vi "RSZVB Calibration Auto.vi"(0 "VISA session":refnum<visa-resource-name>, 1 "Channel (1)":i32=1, 2 "Calibration Kit Name":string, 5 "error in (no error)":errorcluster {"code" format="%.0x"}, 6 "Analyzer Port 1 (1)":i32=1, 7 "Cal Unit Port 1 (1)":i32=1, 8 "Analyzer Port 2 (1)":i32=1, 9 "Cal Unit Port 2 (1)":i32=1, 10 "Analyzer Port 3 (1)":i32=1, 11 "Cal Unit Port 3 (1)":i32=1, 12 "Analyzer Port 4 (1)":i32=1, 13 "Cal Unit Port 4 (1)":i32=1) -> (14 "dup VISA session":refnum<visa-resource-name>, 19 "error out":errorcluster {"code" format="%.0x"})   [LabVIEW 2011]
doc: "This VI selects and initiates a one-port, two-port, three-port or four-port automatic calibration at arbitrary analyzer and calibration unit ports.\n\nNote(s):\n\n(1) Port numbers of the analyzer:\nFor an n-port automatic calibration (n = 1 to 4), n arbitrary (not necessarily consecutive) port numbers must be specified.\n\n(2) Port numbers of the cal unit:\nFor an n-port automatic calibration (n = 1 to 4), n arbitrary (not necessarily consecutive) port numbers must be specified. It is possible to combine arbitrary (not necessarily matching) pairs of analyzer and cal unit ports.\n \nRemote-control command(s):\n[SENSe<Ch>:]CORRection:COLLect:AUTO:PORTs '<file_name>',<analyzer_port_no>,<cal_unit_port_no>{,<analyzer_port_no>,<cal_unit_port_no>}"
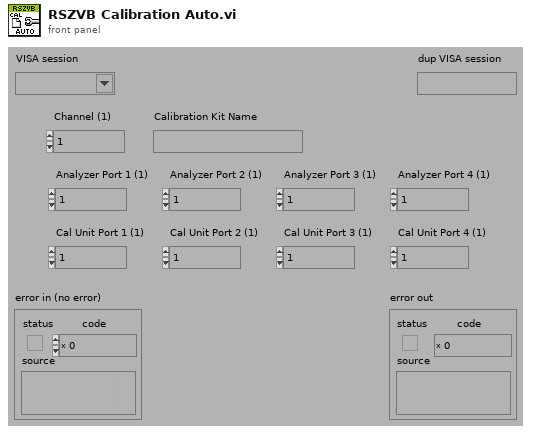
[diagram p1: front panel]
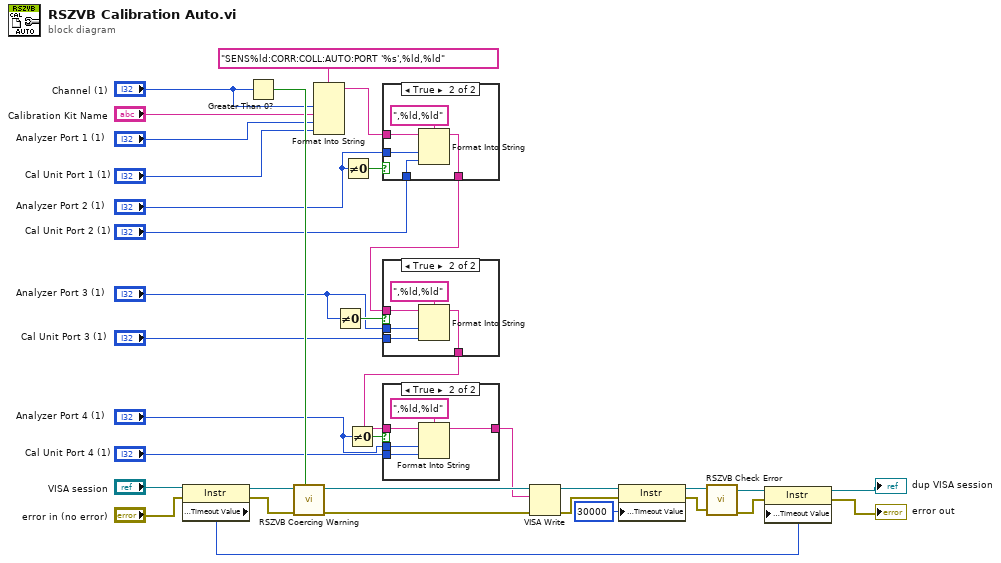
[diagram p0: block diagram]
diagram:
  n1 = property class="Instr"(reference="VISA session", error in="error in (no error)") -> (reference out=w31:refnum<visa-resource-name>, error out=w32:errorcluster, "General Settings:Timeout Value"=w9:u32)
  n2 = Greater Than 0?(x="Channel (1)") -> (x > 0?=w33:bool)
  n3 = call "RSZVB Coercing Warning.vi"("In Range?"=w33, "error in (no error)"=w32, "VISA session"=w31) -> ("error out"=w34:errorcluster, "dup VISA session"=w35:refnum<visa-resource-name>)  [unwired: 7 in]
  n4 = Format Into String(format string="SENS%ld:CORR:COLL:AUTO:PORT '%s',%ld,%ld", "Channel (1)", "Calibration Kit Name", "Analyzer Port 1 (1)", "Cal Unit Port 1 (1)") -> (resulting string=w23:string)  [unwired: 2 in, 1 out]
  n5 = Not Equal To 0?(x="Analyzer Port 3 (1)") -> (x != 0?=w22:bool)
  n6 = Not Equal To 0?(x="Analyzer Port 2 (1)") -> (x != 0?=w24:bool)
  n7 = Not Equal To 0?(x="Analyzer Port 4 (1)") -> (x != 0?=w20:bool)
  n8 = case shown="True" w24 {
    tunnel: w23 -> [w36 w41]
    tunnel: "Analyzer Port 2 (1)" -> [_ w39]
    tunnel: [w36 w38] -> w21
    tunnel: "Cal Unit Port 2 (1)" -> [_ w37]
    frame False {
    }
    frame True {
      n9 = Format Into String(format string=",%ld,%ld", initial string=w41, w39, w37) -> (resulting string=w38:string)  [unwired: 1 in, 1 out]
    }
  }
  n10 = case shown="True" w22 {
    tunnel: w21 -> [w42 w47]
    tunnel: "Analyzer Port 3 (1)" -> [_ w45]
    tunnel: [w42 w44] -> w19
    tunnel: "Cal Unit Port 3 (1)" -> [_ w43]
    frame False {
    }
    frame True {
      n11 = Format Into String(format string=",%ld,%ld", initial string=w47, w45, w43) -> (resulting string=w44:string)  [unwired: 1 in, 1 out]
    }
  }
  n12 = case shown="True" w20 {
    tunnel: w19 -> [w48 w53]
    tunnel: "Analyzer Port 4 (1)" -> [_ w51]
    tunnel: [w48 w50] -> w18
    tunnel: "Cal Unit Port 4 (1)" -> [_ w49]
    frame False {
    }
    frame True {
      n13 = Format Into String(format string=",%ld,%ld", initial string=w53, w51, w49) -> (resulting string=w50:string)  [unwired: 1 in, 1 out]
    }
  }
  n14 = VISA Write(VISA resource name=w35, write buffer=w18, error in (no error)=w34) -> (VISA resource name out=w3:refnum<visa-resource-name>, error out=w2:errorcluster)  [unwired: 1 out]
  n15 = property class="Instr"(reference=w3, error in=w2, "General Settings:Timeout Value"=u32 30000) -> (reference out=w4:refnum<visa-resource-name>, error out=w1:errorcluster)
  n16 = call "RSZVB Check Error.vi"("error in (no error)"=w1, "VISA session"=w4) -> ("error out"=w8:errorcluster, "dup VISA session"=w5:refnum<visa-resource-name>)  [unwired: 8 in]
  n17 = property class="Instr"(reference=w5, error in=w8, "General Settings:Timeout Value"=w9) -> (reference out=→"dup VISA session":refnum<visa-resource-name>, error out=→"error out":errorcluster)
